vi "Read Voltage.vi"(8 "error in (no error)":errorcluster, 11 "DAQmx in":refnum<class "DAQmx.lvclass">) -> (0 "error out":errorcluster, 2 "Voltage":dbl, 3 "DAQmx out":refnum<class "DAQmx.lvclass">)   [LabVIEW 2020, in "DAQmx.lvclass"]
uses:
  DAQmx.lvclass
  DAQmx.lvclass/DAQmx.ctl
  <vilib>/DAQmx/read.llb/DAQmx Read (Analog DBL 1Chan 1Samp).vi
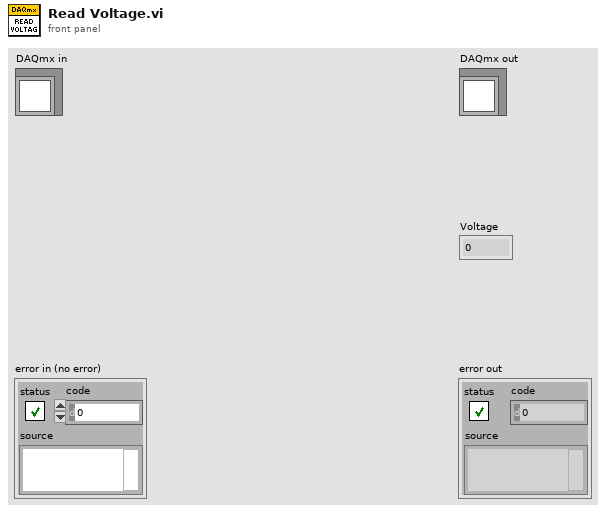
[diagram p1: front panel]
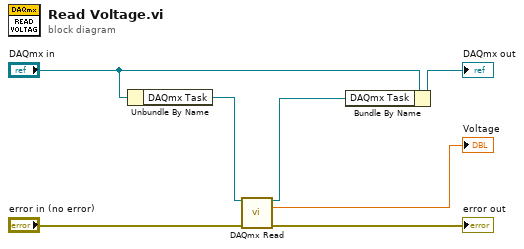
[diagram p0: block diagram]
diagram:
  n1 = Unbundle By Name("DAQmx in") -> ("DAQmx Task"=w3:refnum<k21>)
  n2 = call-poly <vilib>:"DAQmx Read.vi"("task/channels in"=w3, "error in"="error in (no error)") -> ("task out"=w1:refnum<k21>, "data"=→"Voltage":dbl, "error out"=→"error out":errorcluster)  [unwired: 11 in]
  n3 = Bundle By Name(cluster="DAQmx in", "DAQmx Task"=w1) -> (→"DAQmx out":refnum<class "DAQmx.lvclass">)
